vi "Sub Parse File Data.vi"(8 "error in (no error)":errorcluster, 11 "input string":string) -> (0 "error out":errorcluster, 3 "file data":T1)   [LabVIEW 2018, in "Data Parser.lvclass"]
uses:
  Data Parser.lvclass
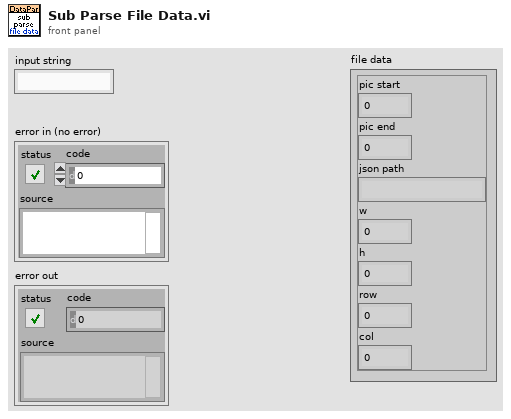
[diagram p1: front panel]
types:
  T1 = cluster{"pic start":i32, "pic end":i32, "json path":string, "w":i32, "h":i32, "row":i32, "col":i32}
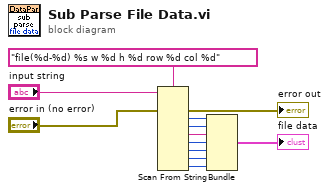
[diagram p0: block diagram]
diagram:
  n1 = Scan From String(format string="file(%d-%d) %s w %d h %d row %d col %d", input string="input string", error in="error in (no error)") -> (error out=→"error out":errorcluster, output 1=w11:i32, output 2=w10:i32, output 3=w9:string, output 4=w8:i32, output 5=w7:i32, output 6=w6:i32, output 7=w5:i32)  [unwired: 8 in, 2 out]
  n2 = Bundle(w11, w10, w9, w8, w7, w6, w5) -> (→"file data":cluster{i32, i32, string, i32, i32, i32, i32})  [unwired: 1 in]
